vi "BRig_dataBlock_T2R.vi"() -> (2 "output_T2R":i32)   [LabVIEW 2014]
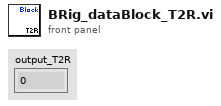
[diagram p1: front panel]
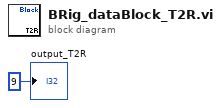
[diagram p0: block diagram]
diagram:
  "output_T2R" <- 9 ("output_iBlock")
